vi "SENS_SWE_DWEL.vi"(0 "VISA IN":refnum<visa-resource-name>, 1 "Dwell Time(sec)":dbl, 5 "error in":errorcluster, 7 "Channel":i32=1) -> (14 "VISA Out":refnum<visa-resource-name>, 19 "error out":errorcluster)   [LabVIEW 2018, in "PNA-X.lvlib"]
doc: "SENSe<cnum>:SWEep:DWELl <num> \n(Read-Write) Sets the dwell time between each sweep point. \nDwell time is ONLY available with SENSe:SWEep:GENeration set to STEPped; It is Not available in \nANALOG. \nSending dwell = 0 is the same as setting SENS:SWE:DWEL:AUTO ON. Sending a dwell time > 0 sets \nSENS:SWE:DWEL:AUTO OFF. \nParameters \n<cnum> Any existing channel number. If unspecified, value is set to 1 \n<num> Dwell time in seconds. \nSee Note \nExamples SENS:SWE:DWEL .1 \nsense2:sweep:dwell min \n1815\n\nQuery Syntax SENSe<cnum>:SWEep:DWELl? \nReturn Type Numeric \nDefault 0 - (Note: dwell time set to 0 is the same as dwell:auto ON)"
uses:
  PNA-X.lvlib
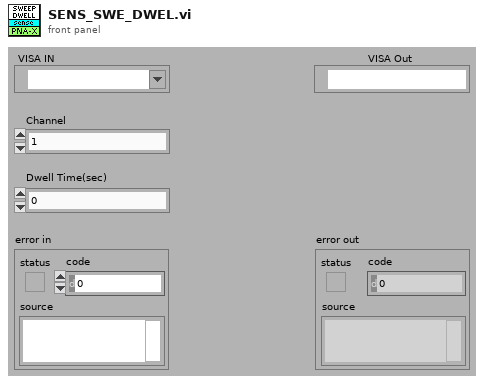
[diagram p1: front panel]
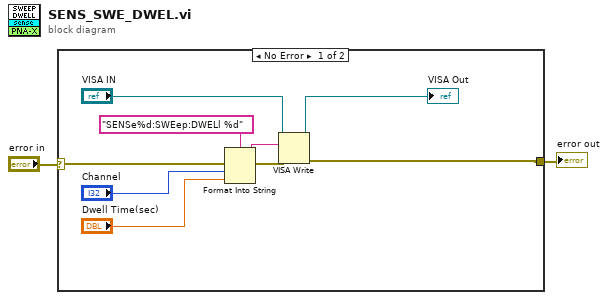
[diagram p0: block diagram]
diagram:
  n1 = case shown="No Error" "error in" {
    selector: "error in" -> [w11 w12]
    tunnel: [w6 w12] -> w1
    frame No Error {
      n2 = Format Into String(format string="SENSe%d:SWEep:DWELl %d" ("Cmdline"), error in=w11, "Channel", "Dwell Time(sec)") -> (resulting string=w9:string, error out=w10:errorcluster)  [unwired: 1 in]
      n3 = VISA Write(VISA resource name="VISA IN", write buffer=w9, error in (no error)=w10) -> (VISA resource name out=→"VISA Out":refnum<visa-resource-name>, error out=w6:errorcluster)  [unwired: 1 out]
    }
    frame Error {
    }
  }
  "error out" <- w1
